vi "PH_Waveplate-GUI_6P.panel.vi"(0 "object ref":refnum<vi>, 5 "error in (no error)":errorcluster) -> (19 "error out":errorcluster)   [LabVIEW 2014, in "PH_Waveplate-GUI_6P.lvlib"]
doc: "By this VI a ross relais can be monitored and switched. \n\nThe indicators \"CLOSED\", \"OPEN\" and \"SWITCH STATE\" show the value of the Beckhoff-Tag: blue indicates bad tag status reference problems, darkgreen false and lightgreen on. If everything is working fine, \"CLOSED\" and \"SWITCH STATE\" should show the same value, while \"OPEN\" has the opposite value. \n\nThe oval button switches the ross relais. It should be in the same state as the \"SWITCH STATE\" indicator. \n\n\"EXIT\" closes the front panel (GUI), while \"Delete Instance\" disconnects and removes the instance from the PCS.\n\nThis VI has no machine safety relevant logig: there is neither a check of internal conclict nor with other objects, for example conflict with other ross relais. Therefore it must be handled with care and should be operated by well educated operators only. It is forseen exclusively for direct operating and testing of the system. \n\nLicense Agreement for this software:\n\nCopyright (C)\nGesellschaft für Schwerionenforschung, GSI\nPlanckstr. 1\n64291 Darmstadt\nGermany\n\nContact: D.Beck@gsi.de \n\nThis program is free software; you can redistribute it and/or modify it under the terms of the GNU General Public License as published by the Free Software Foundation; either version 2 of the license, or (at your option) any later version.\n\nThis program is distributed in the hope that it will be useful, but WITHOUT ANYW ARRANTY; without even the implied warranty of MERCHANTABILITY or FITNESS FOR A PARTICULAR PURPOSE. See the GNU General License for more details (http://www.gnu.org).\n\nGesellschaft für Schwerionenforschung, GSI\nPlanckstr. 1, 64291 Darmstadt, Germany\nFor all questions and ideas contact: M.Richter@gsi.de, H.Brand@gsi.de or D.Beck@gsi.de.\nLast update: 18-DEC-2002"
uses:
  PH_Waveplate-GUI_6P.lvlib
  PH_Basics/PH_Stepmotor_BaseClass/PH_Stepmotor_BaseClass.Axis Settings.ctl
  PH_Basics/PH_Stepmotor_BaseClass/PH_Stepmotor_BaseClass.Motor Type.ctl
  PH_Basics/PH_Stepmotor_BaseClass/PH_Stepmotor_BaseClass.Axis Address.ctl
  PH_Waveplate-GUI_6P.Type.ctl
  PH_Basics/PH_Stepmotor_BaseClass/PH_Stepmotor_BaseClass.Axis Activity.ctl
  PH_Basics/PH_AxisGUI_BaseClass/PH_AxisGUI_BaseClass.Axis GUI Refs.ctl
  PH_Basics/PH_Stepmotor_BaseClass/PH_Stepmotor_BaseClass.Axis Direction.ctl
  PH_Basics/PH_Common/PH_Common.lvlib
  PH_Basics/PH_Stepmotor_BaseClass/PH_Stepmotor_BaseClass.lvlib
  PH_Basics/PH_AxisGUI_BaseClass/PH_AxisGUI_BaseClass.lvlib
  PH_Basics/PH_Class/PH_Class.lvlib
panel:
  out "Status Bar":u32(colorbox)=16777088 caption="Axis1"
  out "Activity":T1
  out "Status":u32(colorbox)=6618880 caption="Axis1"
  in  "Stop":bool caption="SetZero"
  in  "Tab Control":enum32{"Move", "Settings", "Info"}(tab)
  in  "Clear Error":bool
  in  "CLOSE":bool caption="? Steps"
  in  "OPEN":bool caption="? Steps"
  in  "Axis_Target":string="0" caption="Steps"
  out "Meter":cluster{dbl, dbl}(knob)={0.0, 43.865888203726} caption="Polarization Angle" scale=0.0..45.0
  in  "Type":T2 items=["Degrees", "Percent"]
  in  "Axis_Settings":T3={"Sign change"=FALSE, "Width"=0.0, "Calibration"=0.0, "Unit"="Steps", "Motor Type"=enum."Unspecific", "Unit Width"="", "Unit CF"=""} caption="Settings"
  in  "Extend Limits":bool
  in  "Reset":bool
  out "Axis_Information":T5={"Instance"="N/A", "Motor Nr"=0} caption="Sixpack"
  in  "Set Zero":bool
  in  "Delete":bool
  # "PCS"
  # "3.40"
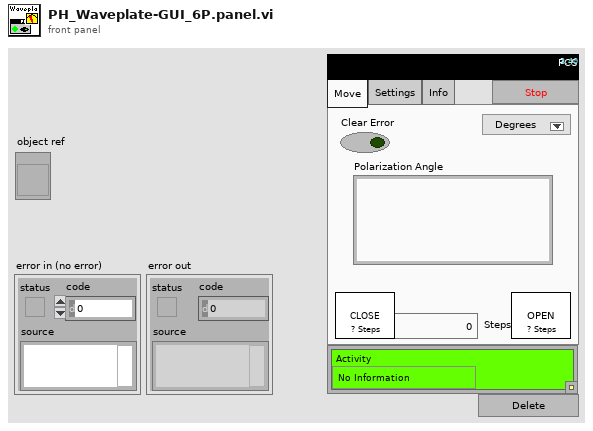
[diagram p1: front panel]
types:
  T1 = typedef "PH_Stepmotor_BaseClass.lvlib/PH_Stepmotor_BaseClass.Axis Activity.ctl" = enum16{"No Information", "stopped", "running", "Failure", "Alarm", "stopped at backward ES", "stopped at foreward ES"}
  T2 = typedef "PH_Waveplate-GUI_6P.lvlib/PH_Waveplate-GUI_6P.Type.ctl" = u16
  T3 = typedef "PH_Stepmotor_BaseClass.lvlib/PH_Stepmotor_BaseClass.Axis Settings.ctl" = cluster{"Sign change":bool, "Width":dbl, "Calibration":dbl, "Unit":string, "Motor Type":T4, "Unit Width":string, "Unit CF":string}
  T4 = typedef "PH_Stepmotor_BaseClass.lvlib/PH_Stepmotor_BaseClass.Motor Type.ctl" = enum16{"Unspecific", "OWIS 49.120.2633", "OWIS 49.060.1033", "OWIS 43.040.2558", "Diamond Motion 2200 series", "OWIS 49.120.266B.MV6", "Calorimeter", "Linear Stage 1", "MICOS VT-80", "MICOS VT-80 S", "Standa Rotstage nt0.95A", "PUF RA 320.200", "PUF RA 800.200", "PUF RA 800.400", "PUF RA 400.50", "1324.nn.800.50", "1324.n9c.800.50", "1324.nn.320.200", "1324.nn.400.200", "1324.nn.800.200", "1324.nn.400.50", "1324.8c9c.800.50", "1324.8c9c.400.200"}
  T5 = typedef "PH_Stepmotor_BaseClass.lvlib/PH_Stepmotor_BaseClass.Axis Address.ctl" = cluster{"Instance":string, "Motor Nr":i32}
  T6 = typedef "PH_AxisGUI_BaseClass.lvlib/PH_AxisGUI_BaseClass.Axis GUI Refs.ctl" = cluster{"Back":refnum<vi>, "Forth":refnum<vi>, "Status":refnum<vi>, "Target":refnum<vi>, "Address":refnum<vi>, "Status Bar":refnum<vi>, "Settings":refnum<vi>, "Activity":refnum<vi>, "Clear Error":refnum<vi>}
  T7 = typedef "PH_Stepmotor_BaseClass.lvlib/PH_Stepmotor_BaseClass.Axis Direction.ctl" = enum16{"forward", "backward"}
  T8 = typedef "PH_Waveplate-GUI_6P.lvlib/PH_Waveplate-GUI_6P.i attribute.ctl" = cluster{"GUI Refs":cluster{"Meter":refnum<vi>, "Extend Limits":refnum<vi>, "Type":refnum<vi>, "Target":refnum<vi>}, "Extend Waveplate Limit":bool, "Type":T2, "Limit":dbl}
  T9 = typedef "PH_AxisGUI_BaseClass.lvlib/PH_AxisGUI_BaseClass.i attribute.ctl" = cluster{"Axes":T10[]}
  T10 = typedef "PH_AxisGUI_BaseClass.lvlib/PH_AxisGUI_BaseClass.Axis Attributes.ctl" = cluster{"Axis GUI Refs":T6, "Address":T5, "Name":string, "Label \"Back\"":string, "Labell \"Forth\"":string, "Moving?":bool}
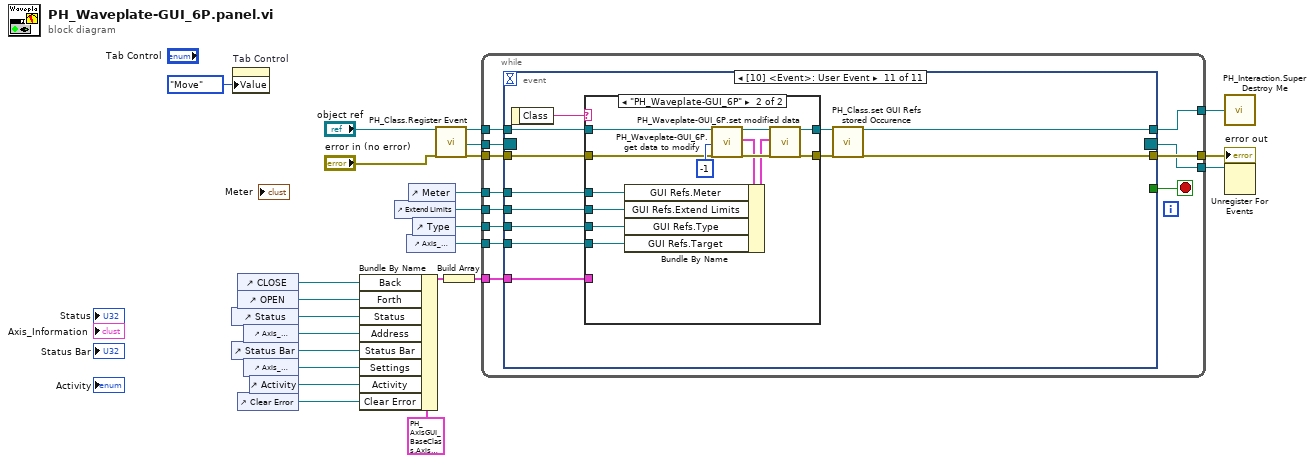
[diagram p0: block diagram]
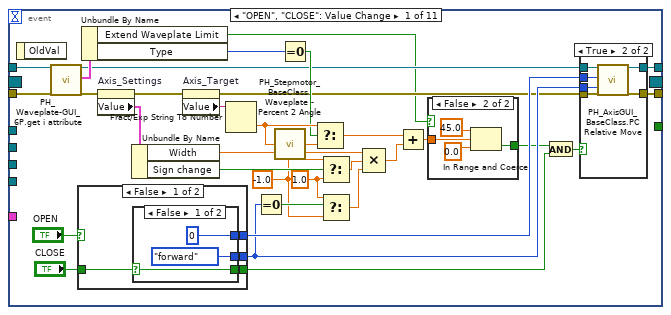
[diagram p2: hidden frame]
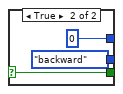
[diagram p4: hidden frame]
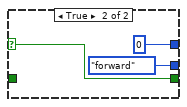
[diagram p5: hidden frame]
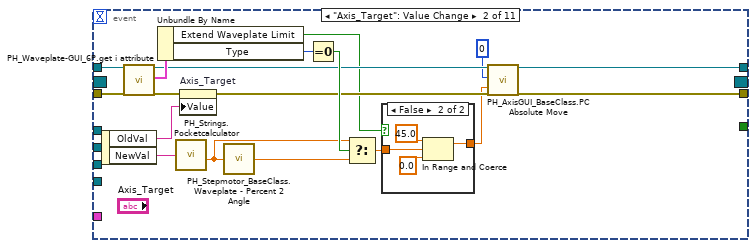
[diagram p7: hidden frame]
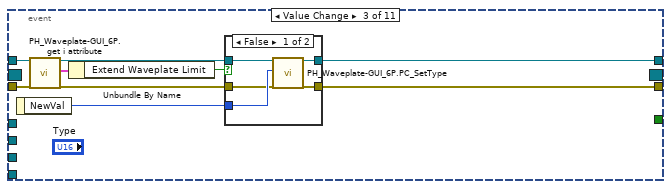
[diagram p9: hidden frame]
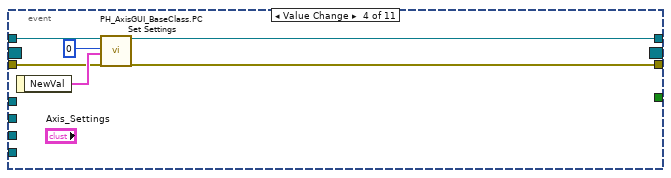
[diagram p11: hidden frame]
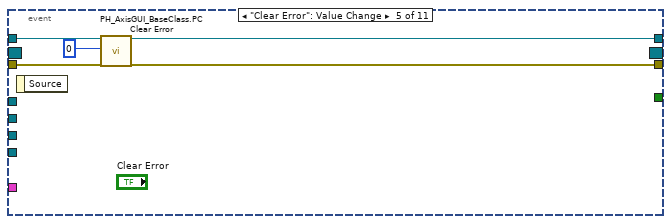
[diagram p12: hidden frame]
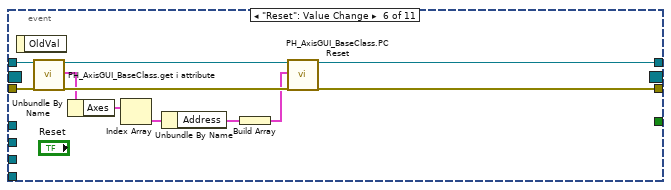
[diagram p13: hidden frame]
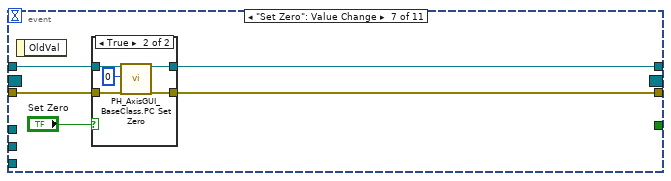
[diagram p14: hidden frame]
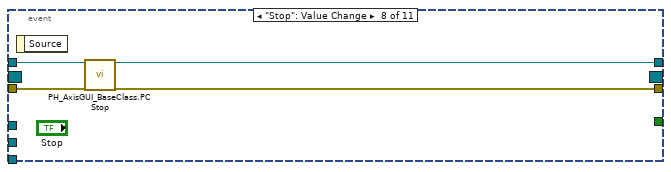
[diagram p16: hidden frame]
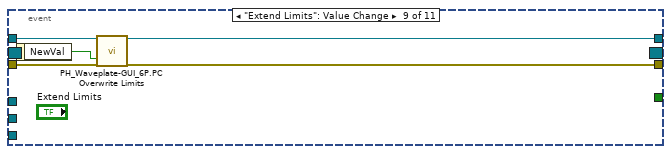
[diagram p17: hidden frame]
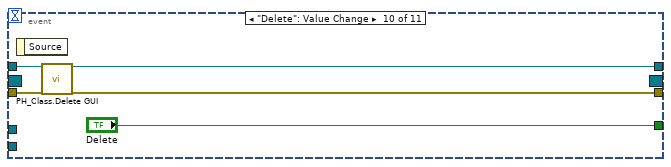
[diagram p18: hidden frame]
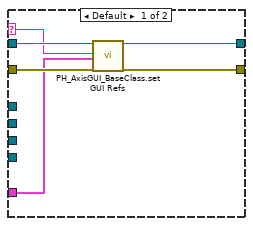
[diagram p19: hidden frame]
diagram:
  n1 = control-ref of="Status"() -> (w15:refnum<vi>)
  n2 = control-ref of="Status Bar"() -> (w13:refnum<vi>)
  n3 = property on="Tab Control" class="TabCtl (strict)"("Value"=enum32{"Move", "Settings", "Info"}."Move" ("Tab Control")) -> ()  [unwired: 2 in, 2 out]
  n4 = control-ref of="CLOSE"() -> (w17:refnum<vi>)
  n5 = control-ref of="OPEN"() -> (w16:refnum<vi>)
  n6 = control-ref of="Clear Error"() -> (w12:refnum<vi>)
  n7 = control-ref of="Axis_Information"() -> (w20:refnum<vi>)
  n8 = control-ref of="Axis_Settings"() -> (w18:refnum<vi>)
  n9 = control-ref of="Activity"() -> (w14:refnum<vi>)
  n10 = Bundle By Name(cluster=T6 {"Back"=refnum, "Forth"=refnum, "Status"=refnum, "Target"=refnum, "Address"=refnum, "Status Bar"=refnum, "Settings"=refnum, "Activity"=refnum, "Clear Error"=refnum} ("GUI Refs"), "Back"=w17, "Forth"=w16, "Status"=w15, "Address"=w20, "Status Bar"=w13, "Settings"=w18, "Activity"=w14, "Clear Error"=w12) -> (w21:T6)
  n11 = control-ref of="Extend Limits"() -> (w6:refnum<vi>)
  n12 = control-ref of="Axis_Target"() -> (w4:refnum<vi>)
  n13 = control-ref of="Meter"() -> (w7:refnum<vi>)
  n14 = control-ref of="Type"() -> (w5:refnum<vi>)
  n15 = call "PH_Class.Register Event.vi"("i ref in"="object ref", "error in (no error)"="error in (no error)") -> ("i ref out"=w10:refnum<vi>, "Event Registration Refnum"=w9:refnum<event-registration>, "error out"=w11:errorcluster)  [unwired: 15 in]
  n16 = Build Array(w21) -> (w3:T6[])
  n17 = while {
    tunnel: w10 -> [w33]
    tunnel: [w32] -> w23
    tunnel: w11 -> [w35]
    tunnel: [w34] -> w24
    tunnel: w9 -> [w31]
    tunnel: [w30] -> w8
    tunnel: w7 -> [w29]
    tunnel: w6 -> [w28]
    tunnel: w5 -> [w27]
    tunnel: w4 -> [w26]
    tunnel: w3 -> [w25]
    stop <- w36 stop-if-true
    n18 = event shown="[10] <Event>: User Event" {
      selector: w31 -> [_ _ _ _ _ _ _ _ _ _ _]
      dyn-events: [_ _ _ _ _ _ _ _ _ _ _] -> w30
      timeout: _ -> [_ _ _ _ _ _ _ _ _ _ _]
      tunnel: [_ _ _ _ _ _ _ _ _ "Delete" _] -> w36
      tunnel: w33 -> [w45 w110 w122 w136 w142 w149 w159 w170 w174 w180 w192]
      tunnel: w35 -> [w46 w112 w124 w135 w141 w148 w158 w169 w173 w181 w190]
      tunnel: [w64 w104 w127 w140 w145 w146 w161 w171 w176 w178 w193] -> w34
      tunnel: [w65 w102 w126 w139 w144 w147 w160 w172 w177 w179 w194] -> w32
      tunnel: w29 -> [_ _ _ _ _ _ _ _ _ _ w187]
      tunnel: w28 -> [_ _ _ _ _ _ _ _ _ _ w186]
      tunnel: w27 -> [_ _ _ _ _ _ _ _ _ _ w185]
      tunnel: w26 -> [_ _ _ _ _ _ _ _ _ _ w184]
      tunnel: w25 -> [_ _ _ _ _ _ _ _ _ _ w183]
      event "OPEN", "CLOSE": Value Change {
        w41 = 1.0 ("t")
        w40 = -1.0 ("f")
        n19 = event-data() -> ()  [unwired: 1 in, 1 out]
        n20 = call "PH_Waveplate-GUI_6P.get i attribute.vi"("i ref in"=w45, "error in (no error)"=w46) -> ("i ref out"=w43:refnum<vi>, "i attribute"=w47:T8, "error out"=w60:errorcluster)  [unwired: 15 in]
        n21 = case shown="False" "OPEN" {
          selector: "OPEN" -> [_ w85]
          tunnel: [w78 0] -> w69
          tunnel: [w77 PH_Stepmotor_BaseClass.Axis_Direction."forward" ("direction")] -> w44
          tunnel: "CLOSE" -> [w76 _]
          tunnel: [w75 w85] -> w68
          frame False {
            n22 = case shown="False" w76 {
              selector: w76 -> [w79 w82]
              tunnel: [0 0] -> w78
              tunnel: [PH_Stepmotor_BaseClass.Axis_Direction."forward" ("direction") PH_Stepmotor_BaseClass.Axis_Direction."backward" ("direction")] -> w77
              tunnel: [w79 w82] -> w75
              frame False {
              }
              frame True {
              }
            }
          }
          frame True {
          }
        }
        n23 = Unbundle By Name(w47) -> ("Extend Waveplate Limit"=w37:bool, "Type"=w48:T2)
        n24 = property on="Axis_Settings" class="Clust (strict)"(error in=w60) -> (error out=w61:errorcluster, "Value"=w55:T3)  [unwired: 1 in, 1 out]
        n25 = Unbundle By Name(w55) -> ("Width"=w56:dbl, "Sign change"=w57:bool)
        n26 = property on="Axis_Target" class="Str"(error in=w61) -> (error out=w42:errorcluster, "Value"=w54:string)  [unwired: 1 in, 1 out]
        n27 = Fract/Exp String To Number(string=w54) -> (number=w51:dbl)  [unwired: 3 in, 1 out]
        n28 = Equal To 0?(x=w44) -> (x = 0?=w62:bool)
        n29 = call "PH_Stepmotor_BaseClass.Waveplate - Percent 2 Angle.vi"("rel. Intensity [%]"=w51) -> ("Angle [°]"=w50:dbl)
        n30 = Equal To 0?(x=w48) -> (x = 0?=w49:bool)
        n31 = Select(t=w51, s=w49, f=w50) -> (s? t:f=w52:dbl)
        n32 = Select(t=w40, s=w57, f=w41) -> (s? t:f=w59:dbl)
        n33 = Select(t=w41, s=w62, f=w40) -> (s? t:f=w63:dbl)
        n34 = Compound Arithmetic op=MULTIPLY(w56, w59, w63) -> (w58:dbl)
        n35 = Add(x=w52, y=w58) -> (x+y=w53:dbl)
        n36 = case shown="False" w37 {
          selector: w37 -> [w70 _]
          tunnel: w53 -> [_ w74]
          tunnel: [w70 w71] -> w38
          frame True {
          }
          frame False {
            n37 = In Range and Coerce(upper limit=45.0, x=w74, lower limit=0.0) -> (In Range?=w71:bool)  [unwired: 1 out]
          }
        }
        n38 = And(x=w38, y=w68) -> (x .and. y?=w39:bool)
        n39 = case shown="True" w39 {
          tunnel: w42 -> [w88 w95]
          tunnel: w43 -> [w89 w94]
          tunnel: w44 -> [_ w93]
          tunnel: [w89 w92] -> w65
          tunnel: [w88 w91] -> w64
          tunnel: w69 -> [_ w90]
          frame False {
          }
          frame True {
            n40 = call "PH_AxisGUI_BaseClass.PC Relative Move.vi"("i ref in"=w94, "Axis"=w90, "direction"=w93, "error in"=w95) -> ("i ref out"=w92:refnum<vi>, "error out"=w91:errorcluster)  [unwired: 14 in]
          }
        }
      }
      event "Axis_Target": Value Change {
        n41 = event-data() -> ("OldVal"=w97:string, "NewVal"=w113:string)  [unwired: 1 in]
        n42 = call "PH_Waveplate-GUI_6P.get i attribute.vi"("i ref in"=w110, "error in (no error)"=w112) -> ("i ref out"=w103:refnum<vi>, "i attribute"=w109:T8, "error out"=w111:errorcluster)  [unwired: 15 in]
        n43 = Unbundle By Name(w109) -> ("Extend Waveplate Limit"=w96:bool, "Type"=w108:T2)
        n44 = call "PH_Strings.Pocketcalculator.vi"("Input"=w113) -> ("Double"=w98:dbl)  [unwired: 3 out]
        n45 = property on="Axis_Target" class="Str"(error in=w111, "Value"=w97) -> (error out=w105:errorcluster)  [unwired: 1 in, 1 out]
        n46 = call "PH_Stepmotor_BaseClass.Waveplate - Percent 2 Angle.vi"("rel. Intensity [%]"=w98) -> ("Angle [°]"=w106:dbl)
        n47 = Equal To 0?(x=w108) -> (x = 0?=w107:bool)
        n48 = Select(t=w98, s=w107, f=w106) -> (s? t:f=w101:dbl)
        n49 = case shown="False" w96 {
          tunnel: w101 -> [w114 w118]
          tunnel: [w114 w117] -> w99
          frame True {
          }
          frame False {
            n50 = In Range and Coerce(upper limit=45.0, x=w118, lower limit=0.0) -> (coerced(x)=w117:dbl)  [unwired: 1 out]
          }
        }
        n51 = call "PH_AxisGUI_BaseClass.PC Absolute Move.vi"("i ref in"=w103, "Axis"=0, "Position [Units]"=w99, "error in"=w105) -> ("i ref out"=w102:refnum<vi>, "error out"=w104:errorcluster)  [unwired: 14 in]
      }
      event Value Change {
        n52 = event-data() -> ("NewVal"=w125:T2)  [unwired: 1 in]
        n53 = call "PH_Waveplate-GUI_6P.get i attribute.vi"("i ref in"=w122, "error in (no error)"=w124) -> ("i ref out"=w121:refnum<vi>, "i attribute"=w120:T8, "error out"=w123:errorcluster)  [unwired: 15 in]
        n54 = Unbundle By Name(w120) -> ("Extend Waveplate Limit"=w119:bool)
        n55 = case shown="False" w119 {
          tunnel: [w132 w133] -> w127
          tunnel: [w131 w134] -> w126
          tunnel: w125 -> [w130 _]
          tunnel: w123 -> [w129 w133]
          tunnel: w121 -> [w128 w134]
          frame False {
            n56 = call "PH_Waveplate-GUI_6P.PC_SetType.vi"("VI in"=w128, "Type"=w130, "error in"=w129) -> ("VI out"=w131:refnum<vi>, "error out"=w132:errorcluster)  [unwired: 15 in]
          }
          frame True {
          }
        }
      }
      event Value Change {
        n57 = event-data() -> ("NewVal"=w138:T3)  [unwired: 1 in]
        n58 = call "PH_AxisGUI_BaseClass.PC Set Settings.vi"("VI in"=w136, "Axis"=0, "NewVal"=w138, "error in (no error)"=w135) -> ("VI out"=w139:refnum<vi>, "error out"=w140:errorcluster)  [unwired: 14 in]
      }
      event "Clear Error": Value Change {
        n59 = event-data() -> ()  [unwired: 1 in, 1 out]
        n60 = call "PH_AxisGUI_BaseClass.PC Clear Error.vi"("i ref in"=w142, "Axis"=0, "error in"=w141) -> ("i ref out"=w144:refnum<vi>, "error out"=w145:errorcluster)  [unwired: 15 in]
      }
      event "Reset": Value Change {
        n61 = event-data() -> ()  [unwired: 1 in, 1 out]
        n62 = call "PH_AxisGUI_BaseClass.get i attribute.vi"("i ref in"=w149, "error in (no error)"=w148) -> ("i ref out"=w155:refnum<vi>, "i attribute"=w154:T9, "error out"=w156:errorcluster)  [unwired: 15 in]
        n63 = Unbundle By Name(w154) -> ("Axes"=w153:T10[])
        n64 = Index Array(array=w153) -> (element=w152:T10)  [unwired: 1 in]
        n65 = Unbundle By Name(w152) -> ("Address"=w151:T5)
        n66 = Build Array(w151) -> (w150:T5[])
        n67 = call "PH_AxisGUI_BaseClass.PC Reset.vi"("i ref in"=w155, "Addresses"=w150, "error in"=w156) -> ("i ref out"=w147:refnum<vi>, "error out"=w146:errorcluster)  [unwired: 15 in]
      }
      event "Set Zero": Value Change {
        n68 = event-data() -> ()  [unwired: 1 in, 1 out]
        n69 = case shown="True" "Set Zero" {
          tunnel: [w162 w168] -> w161
          tunnel: [w163 w167] -> w160
          tunnel: w159 -> [w163 w166]
          tunnel: w158 -> [w162 w165]
          frame False {
          }
          frame True {
            n70 = call "PH_AxisGUI_BaseClass.PC Set Zero.vi"("VI in"=w166, "Axis"=0, "error in (no error)"=w165) -> ("VI out"=w167:refnum<vi>, "error out"=w168:errorcluster)  [unwired: 15 in]
          }
        }
      }
      event "Stop": Value Change {
        n71 = event-data() -> ()  [unwired: 1 in, 1 out]
        n72 = call "PH_AxisGUI_BaseClass.PC Stop.vi"("VI in"=w170, "error in (no error)"=w169) -> ("VI out"=w172:refnum<vi>, "error out"=w171:errorcluster)  [unwired: 16 in]
      }
      event "Extend Limits": Value Change {
        n73 = event-data() -> ("NewVal"=w175:bool)  [unwired: 1 in]
        n74 = call "PH_Waveplate-GUI_6P.PC Overwrite Limits.vi"("i ref in"=w174, "Overwrite Limits?"=w175, "error in"=w173) -> ("i ref out"=w177:refnum<vi>, "error out"=w176:errorcluster)  [unwired: 15 in]
      }
      event "Delete": Value Change {
        n75 = event-data() -> ()  [unwired: 1 in, 1 out]
        n76 = call "PH_Class.Delete GUI.vi"("VI in"=w180, "error in (no error)"=w181) -> ("VI out"=w179:refnum<vi>, "error out"=w178:errorcluster)  [unwired: 16 in]
      }
      event User Event {
        n77 = event-data() -> ("Class"=w188:string)  [unwired: 1 in]
        n78 = case shown="\"PH_Waveplate-GUI_6P\"" w188 {
          selector: w188 -> [w196 _]
          tunnel: w192 -> [w200 w209]
          tunnel: [w198 w207] -> w191
          tunnel: w190 -> [w199 w206]
          tunnel: [w197 w205] -> w189
          tunnel: w187 -> [_ w204]
          tunnel: w186 -> [_ w203]
          tunnel: w185 -> [_ w202]
          tunnel: w184 -> [_ w201]
          tunnel: w183 -> [w195 _]
          frame Default {
            n79 = call "PH_AxisGUI_BaseClass.set GUI Refs.vi"("i ref in"=w200, "Class"=w196, "Axis GUI Base Class Refs"=w195, "error in"=w199) -> ("i ref out"=w198:refnum<vi>, "error out"=w197:errorcluster)  [unwired: 14 in]
          }
          frame "PH_Waveplate-GUI_6P" {
            n80 = call "PH_Waveplate-GUI_6P.get data to modify.vi"("i ref in"=w209, "ms timeout (10000)"=-1, "error in (no error)"=w206) -> ("i ref out"=w213:refnum<vi>, "i attribute"=w211:T8, "error out"=w212:errorcluster)  [unwired: 13 in, 1 out]
            n81 = Bundle By Name(cluster=w211, "GUI Refs.Meter"=w204, "GUI Refs.Extend Limits"=w203, "GUI Refs.Type"=w202, "GUI Refs.Target"=w201) -> (w210:T8)
            n82 = call "PH_Waveplate-GUI_6P.set modified data.vi"("i ref in"=w213, "i attribute"=w210, "error in (no error)"=w212) -> ("i ref out"=w207:refnum<vi>, "error out"=w205:errorcluster)  [unwired: 15 in]
          }
        }
        n83 = call "PH_Class.set GUI Refs stored Occurence.vi"("i ref in"=w191, "error in (no error)"=w189) -> ("i ref out"=w194:refnum<vi>, "error out"=w193:errorcluster)  [unwired: 16 in]
      }
    }
  }
  "error out" <- w24
  n84 = call "PH_Interaction.Super Destroy Me.vi"("i ref out"=w23) -> ()
  n85 = Unregister For Events(event registration refnum=w8) -> ()  [unwired: 1 in, 1 out]
